vi "TransformObjectPosition.vi"(4 "Pixel size Y":dbl, 6 "Image time":dbl, 8 "error in (no error)":errorcluster, 9 "Pixel size X":dbl, 10 "Objects (pixel)":T1(array[cluster]), 11 "Spacetime cluster":T2) -> (0 "error out":errorcluster, 1 "Focus out":dbl, 2 "Y out":dbl, 3 "X out":dbl)   [LabVIEW 2012]
panel:
  out "Y center":dbl(graph)
  out "X center":dbl(graph)
  out "X stage":dbl(graph)
  out "Y stage":dbl(graph)
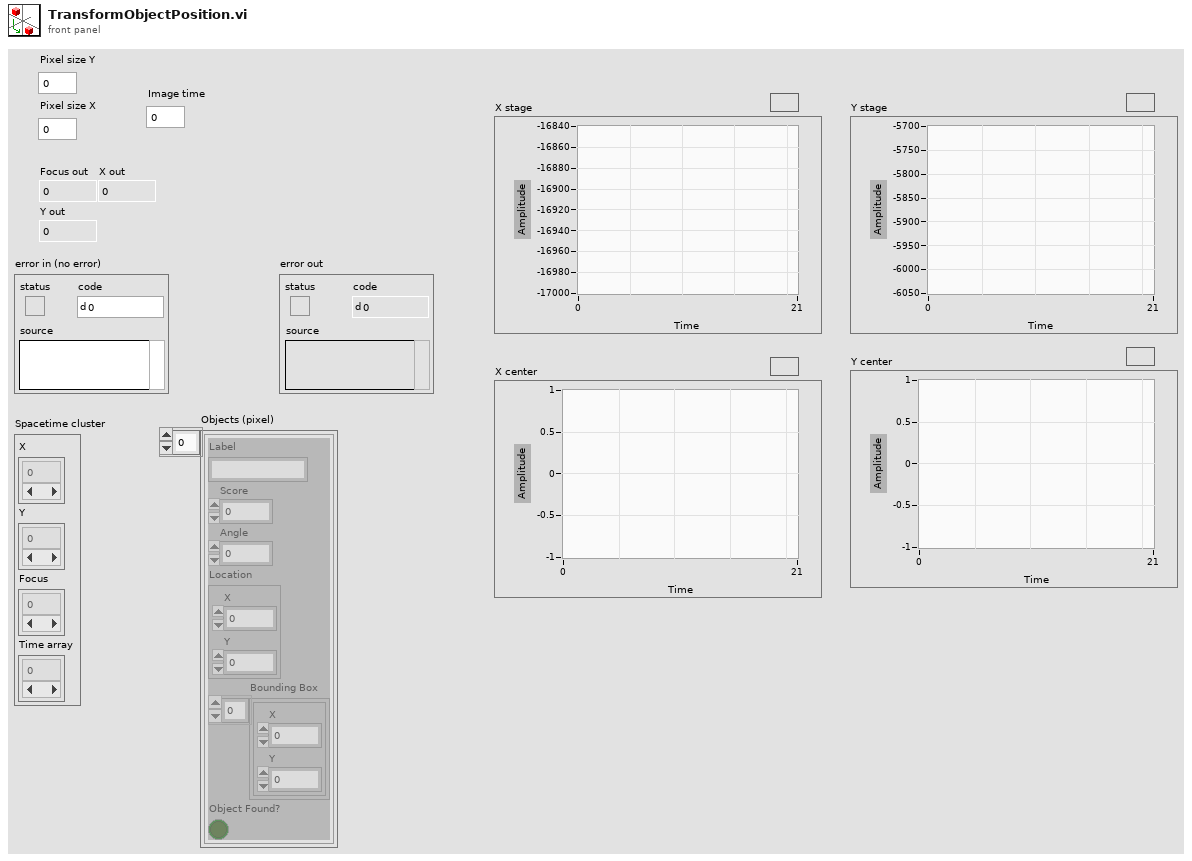
[diagram p1: front panel]
types:
  T1 = cluster{"Label":string, "Score":i32, "Angle":dbl, "Location":cluster{"X":dbl, "Y":dbl}, "Bounding Box":cluster{"X":dbl, "Y":dbl}[], "Object Found?":bool}[]
  T2 = cluster{"X":dbl[], "Y":dbl[], "Focus":dbl[], "Time array":dbl[]}
  T3 = cluster{"Label":string, "Score":i32, "Angle":dbl, "Location":cluster{"X":dbl, "Y":dbl}, "Bounding Box":cluster{"X":dbl, "Y":dbl}[], "Object Found?":bool}
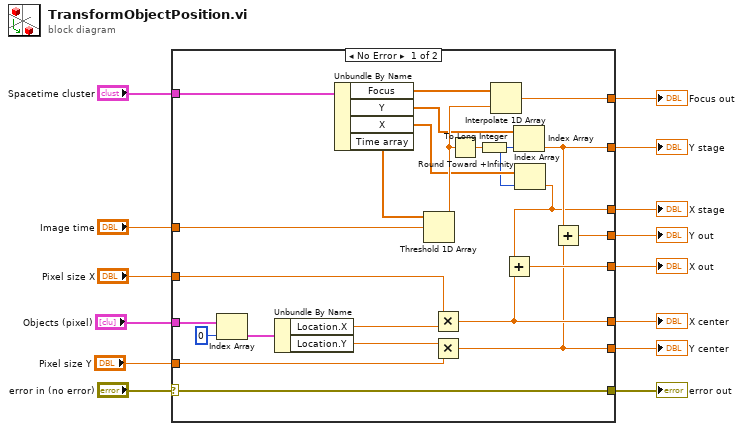
[diagram p0: block diagram]
diagram:
  n1 = case shown="No Error" "error in (no error)" {
    selector: "error in (no error)" -> [w30 w39]
    tunnel: [w30 w39] -> w13
    tunnel: "Objects (pixel)" -> [w38 _]
    tunnel: "Pixel size X" -> [w35 _]
    tunnel: "Image time" -> [w34 _]
    tunnel: [w33 _] -> w10
    tunnel: [w32 _] -> w9
    tunnel: [w31 _] -> w8
    tunnel: "Spacetime cluster" -> [w29 _]
    tunnel: [w23 _] -> w6
    tunnel: [w20 _] -> w5
    tunnel: [w18 _] -> w4
    tunnel: [w17 _] -> w3
    tunnel: "Pixel size Y" -> [w15 _]
    frame No Error {
      n2 = Index Array(array=w38, index=0) -> (element=w36:T3)
      n3 = Unbundle By Name(w36) -> ("Location.X"=w19:dbl, "Location.Y"=w16:dbl)
      n4 = Unbundle By Name(w29) -> ("Focus"=w28:dbl[], "Y"=w24:dbl[], "X"=w22:dbl[], "Time array"=w27:dbl[])
      n5 = Threshold 1D Array(2:w34, 3:w27) -> (0:w26:dbl)  [unwired: 1 in]
      n6 = Multiply(x=w35, y=w19) -> (x*y=w18:dbl)
      n7 = Multiply(x=w16, y=w15) -> (x*y=w17:dbl)
      n8 = Round Toward +Infinity(x=w26) -> (ceil(x): smallest int >= x=w25:dbl)
      n9 = To Long Integer(number=w25) -> (32bit integer=w21:i32)
      n10 = Interpolate 1D Array(1:w26, 2:w28) -> (0:w33:dbl)
      n11 = Index Array(array=w24, index=w21) -> (element=w23:dbl)
      n12 = Index Array(array=w22, index=w21) -> (element=w20:dbl)
      n13 = Add(x=w20, y=w18) -> (x+y=w31:dbl)
      n14 = Add(x=w23, y=w17) -> (x+y=w32:dbl)
    }
    frame Error {
    }
  }
  "error out" <- w13
  "Focus out" <- w10
  "Y out" <- w9
  "X out" <- w8
  "Y stage" <- w6
  "X stage" <- w5
  "X center" <- w4
  "Y center" <- w3
